vi "IMIC_SetYMoving.vi"(0 "X-speed":dbl, 5 "handle":u64) -> (1 "handle out":u64, 2 "output param":T1(ring))   [LabVIEW 2011]
uses:
  tillimic32.dll
panel:
  # "never used"
  # "runs simultanous with xmove"
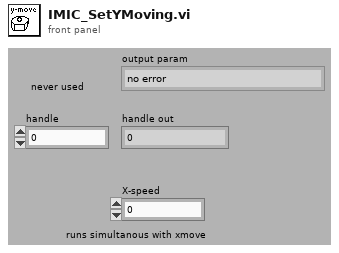
[diagram p1: front panel]
types:
  T1 = enum16{"no error", "missing axis", "missing Z axis", "missing Filter", "iMic not initialized", "no property", "wrong handle", "protocol not finished", "user parameter to long (>32 bits)", "no user parameter handle", "failed to open comport", "failed to initialize"}
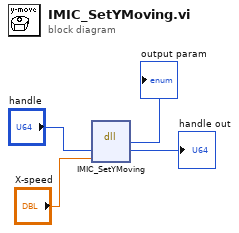
[diagram p0: block diagram]
diagram:
  n1 = dll-call lib="D:/Colibri/Drivers/TILLPhotonics/tillimic*.*" fn="IMIC_SetYMoving"("handle"="handle", "speed"="X-speed") -> ("return type"=→"output param":i32, "handle"=→"handle out":u64)  [unwired: 4 in, 2 out]
